vi "(SubVI)Control Data_Save or Load Control Value.vi"(5 "Val(Sgnl)":bool, 6 "Common? (f)":bool, 7 "Function":T1, 8 "error in (no error)":errorcluster caption="에러 입력(에러 없음)", 9 "Path":path, 10 "Use Default Path (t)":bool=TRUE, 11 "Control Ref":refnum<vi>[](array[refnum])) -> (0 "error out":errorcluster caption="에러 출력")   [LabVIEW 2020]
uses:
  Controls/(Ctrl)Control Data_Save or Load Control Data_Function.ctl
  Variables/(Var)System Variables.vi
  <vilib>/Utility/config.llb/Write Key (String).vi
  <vilib>/Utility/config.llb/Read Key (String).vi
  <vilib>/Utility/config.llb/NI_LVConfig.lvlib
panel:
  # "(SubVI)Save or Load Control Value.vi By hspark\n\nDescription : 컨트롤/인디케이터의 현재 값을 저장하거나, 저장된 값을 불러오는 VI\n\nInput : \n1. Control Ref : 저장 또는 불러오기를 수행할 컨트롤의 참조 배열\n2. Use Default Path : Ture 입력 시 지정된 기본 경로에 저장, False 입력 시 Path로 입력된 경로에 저장\n3. Path : Use Default Path에 False 입력 시 입력 경로 사용\n4. Function : 저장 또는 불러오기 동작 입력\n5. Val(Sgnl) : True 입력 시 값(신호) 프로퍼티로 값을 입력함 (불러오기 시에만 해당)\n6. Common?: False 입력 시 Default Path에 Chip Type을 추가한 경로 사용\n\nOutput : \n\nLabVIEW Version : 2020 SP1 이상\n\nNote :\nINI 파일 형식을 사용함\n섹션 : 컨트롤/인디케이터의 소유자 VI\n키 : 컨트롤의 라벨\n값 : 배리언트 변환 후 패턴화\n\n* 컨트롤/인디케이터 라벨 또는 VI 이름 변경 시 저장된 값 불러오기 안됨\n\nUpdate : 2022.01.06"
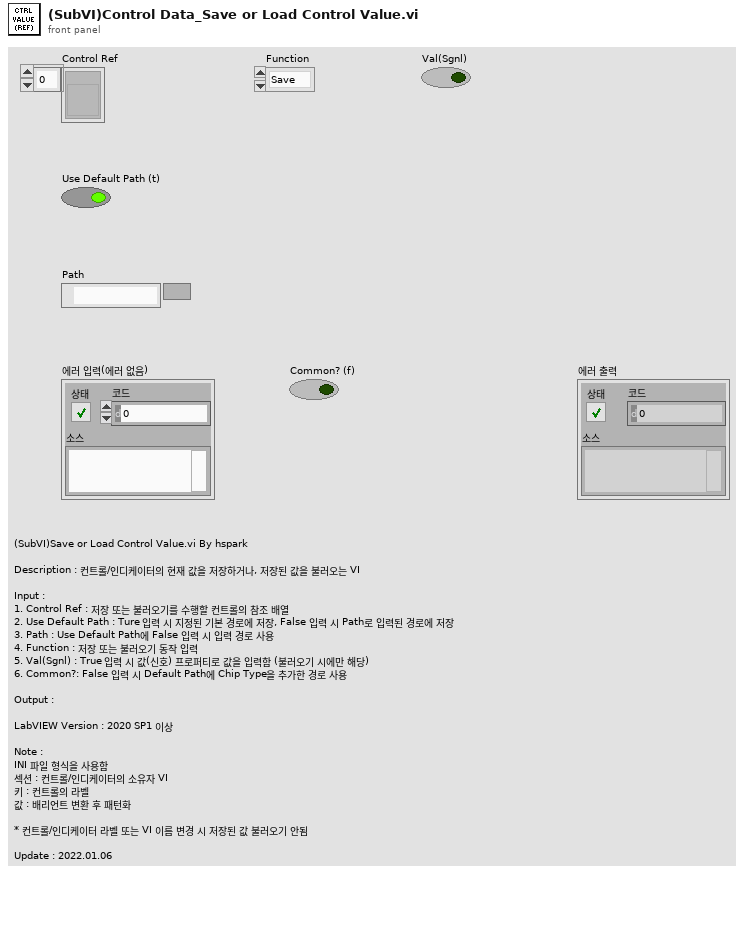
[diagram p1: front panel]
types:
  T1 = typedef "(Ctrl)Control Data_Save or Load Control Data_Function.ctl" = enum16{"Save", "Load"}
  T2 = typedef "Haptic IC.lvclass/(Ctrl)IC Type.ctl" = enum8{"DW7800", "DW7802", "DW7912", "DW7914"}
  T3 = typedef "NI_LVConfig.lvlib/Config Data RefNum.ctl" = refnum<k1>
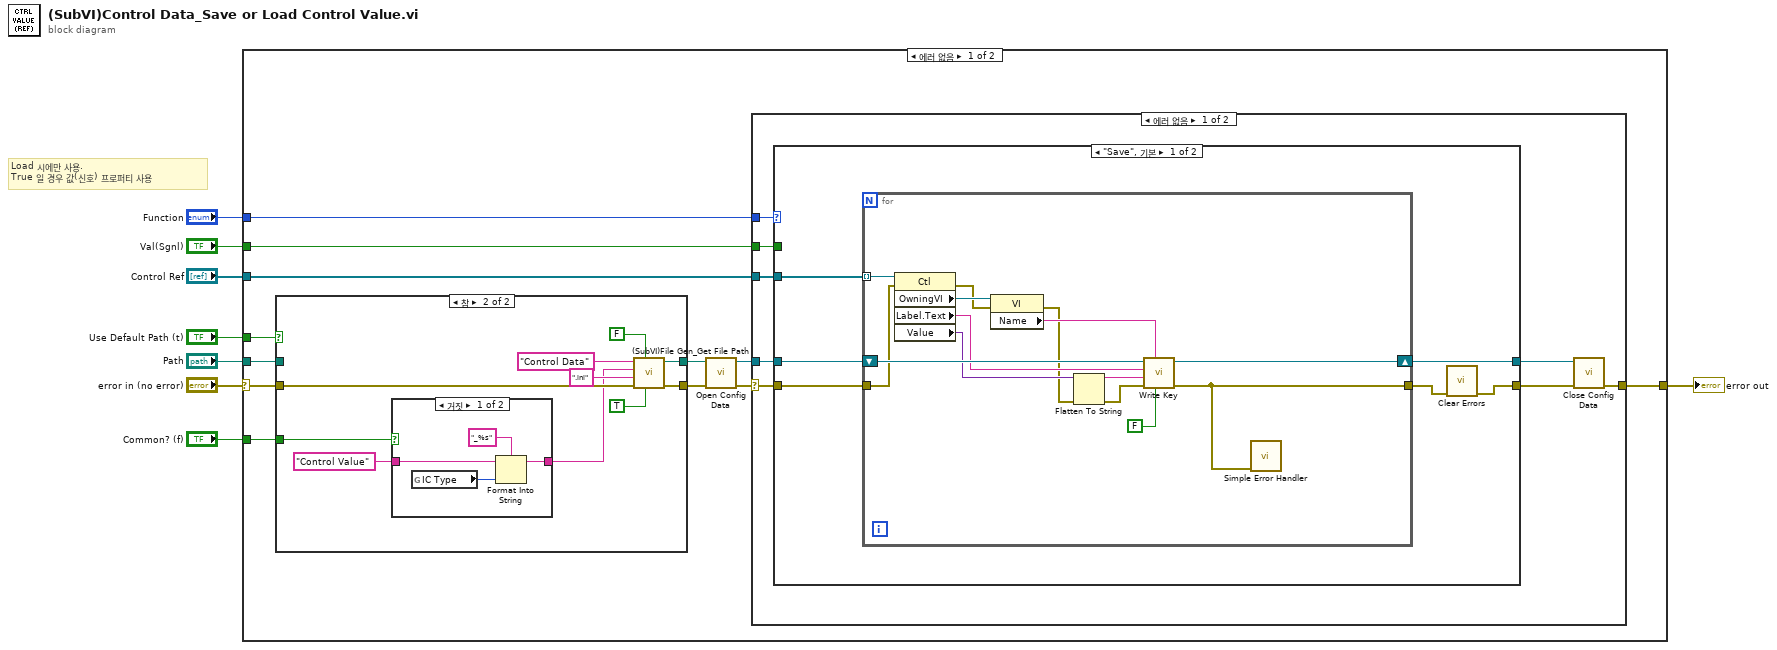
[diagram p0: block diagram]
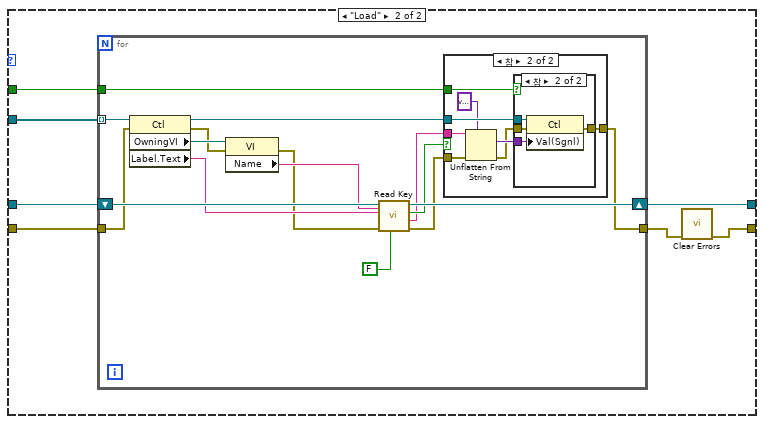
[diagram p4: hidden frame]
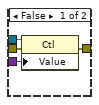
[diagram p6: hidden frame]
diagram:
  # "Load 시에만 사용.\nTrue 일 경우 값(신호) 프로퍼티 사용"
  n1 = case shown="에러 없음" "error in (no error)" {
    selector: "error in (no error)" -> [w14 w107]
    tunnel: [w18 w107] -> w7
    tunnel: "Function" -> [w17 _]
    tunnel: "Control Ref" -> [w16 _]
    tunnel: "Val(Sgnl)" -> [w15 _]
    tunnel: "Use Default Path (t)" -> [w11 _]
    tunnel: "Path" -> [w10 _]
    tunnel: "Common? (f)" -> [w9 _]
    frame No Error {
      n2 = case shown="참" w11 {
        tunnel: w14 -> [w21 w30]
        tunnel: [w21 w29] -> w13
        tunnel: [w22 w28] -> w12
        tunnel: w10 -> [w22 _]
        tunnel: w9 -> [_ w26]
        frame False {
        }
        frame True {
          n3 = case shown="거짓" w26 {
            tunnel: "Control Value" -> [w35 w37]
            tunnel: [w33 w37] -> w24
            frame False {
              n4 = global read "(Var)System Variables.vi" "IC Type"() -> (w34:T2)
              n5 = Format Into String(format string="_%s" ("포맷 문자열"), initial string=w35, w34) -> (resulting string=w33:string)  [unwired: 1 in, 1 out]
            }
            frame True {
            }
          }
          n6 = call "(SubVI)File Gen_Get File Path.vi"("Common?"=TRUE ("Common? (f)"), "Use Timestamp"=FALSE, "error in (no error)"=w30, "File Extension (.txt)"=".ini", "File Name"=w24, "Folder Name"="Control Data") -> ("error out"=w29:errorcluster, "Path"=w28:path)  [unwired: 3 in, 1 out]
        }
      }
      n7 = call <vilib>:"Open Config Data.vi"("error in (no error)"=w13, "configuration file path"=w12) -> ("error out"=w19:errorcluster, "refnum"=w20:T3)  [unwired: 7 in, 1 out]
      n8 = case shown="에러 없음" w19 {
        selector: w19 -> [w43 w106]
        tunnel: w17 -> [w45 _]
        tunnel: w20 -> [w44 _]
        tunnel: [w41 w106] -> w18
        tunnel: w16 -> [w40 _]
        tunnel: w15 -> [w38 _]
        frame No Error {
          n9 = case shown="\"Save\", 기본" w45 {
            tunnel: w44 -> [w51 w72]
            tunnel: w43 -> [w49 w70]
            tunnel: [w46 w67] -> w42
            tunnel: w40 -> [w50 w71]
            tunnel: [w48 w69] -> w39
            tunnel: w38 -> [_ w66]
            frame "Save", Default {
              n10 = for {
                tunnel: w50 -> [w65] mode=indexing
                tunnel: w49 -> [w61]
                shift-right: [w54] -> w48
                shift-left: w51 -> [w64]
                tunnel: [w52] -> w47
                n11 = property class="Ctl"(reference=w65, error in=w61) -> (error out=w62:errorcluster, "OwningVI"=w63:refnum<vi>, "Label.Text"=w59:string, "Value"=w58:variant)  [unwired: 1 out]
                n12 = property class="VI"(reference=w63, error in=w62) -> (error out=w57:errorcluster, "Name"=w60:string)  [unwired: 1 out]
                n13 = Flatten To String(anything=w58, error in (no error)=w57) -> (data string=w56:string, error out=w55:errorcluster)  [unwired: 2 in, 1 out]
                n14 = call-poly <vilib>:"Write Key.vi"("write raw string? (F)"=FALSE, "section"=w60, "error in (no error)"=w55, "value"=w56, "key"=w59, "refnum"=w64) -> ("error out"=w52:errorcluster, "refnum out"=w54:T3)  [unwired: 3 in, 1 out]
                n15 = call <vilib>:"Simple Error Handler.vi"("error in (no error)"=w52) -> ()  [unwired: 4 in, 5 out]
              }
              n16 = call <vilib>:"Clear Errors.vi"("error in (no error)"=w47) -> ("error out"=w46:errorcluster)  [unwired: 5 in, 1 out]
            }
            frame "Load" {
              n17 = for {
                tunnel: w71 -> [w88] mode=indexing
                tunnel: w70 -> [w84]
                shift-right: [w81] -> w69
                shift-left: w72 -> [w87]
                tunnel: [w73] -> w68
                tunnel: w66 -> [w74]
                n18 = property class="Ctl"(reference=w88, error in=w84) -> (reference out=w76:refnum<vi>, error out=w85:errorcluster, "OwningVI"=w86:refnum<vi>, "Label.Text"=w82:string)
                n19 = property class="VI"(reference=w86, error in=w85) -> (error out=w80:errorcluster, "Name"=w83:string)  [unwired: 1 out]
                n20 = call-poly <vilib>:"Read Key.vi"("read raw string? (F)"=FALSE ("write raw string? (F)"), "section"=w83, "error in (no error)"=w80, "key"=w82, "refnum"=w87) -> ("error out"=w75:errorcluster, "value"=w77:string, "found?"=w78:bool, "refnum out"=w81:T3)  [unwired: 3 in]
                n21 = case shown="참" w78 {
                  tunnel: w77 -> [_ w96]
                  tunnel: w76 -> [_ w97]
                  tunnel: w75 -> [w89 w93]
                  tunnel: [w89 w91] -> w73
                  tunnel: w74 -> [_ w90]
                  frame False {
                  }
                  frame True {
                    n22 = Unflatten From String(type=variant ("값"), binary string=w96, error in (no error)=w93) -> (value=w95:variant, error out=w92:errorcluster)  [unwired: 2 in, 1 out]
                    n23 = case shown="참" w90 {
                      tunnel: w97 -> [w101 w105]
                      tunnel: w95 -> [w100 w104]
                      tunnel: w92 -> [w99 w103]
                      tunnel: [w98 w102] -> w91
                      frame False {
                        n24 = property class="Ctl"(reference=w101, error in=w99, "Value"=w100) -> (error out=w98:errorcluster)  [unwired: 1 out]
                      }
                      frame True {
                        n25 = property class="Ctl"(reference=w105, error in=w103, "Val(Sgnl)"=w104) -> (error out=w102:errorcluster)  [unwired: 1 out]
                      }
                    }
                  }
                }
              }
              n26 = call <vilib>:"Clear Errors.vi"("error in (no error)"=w68) -> ("error out"=w67:errorcluster)  [unwired: 5 in, 1 out]
            }
          }
          n27 = call <vilib>:"Close Config Data.vi"("error in (no error)"=w42, "refnum"=w39) -> ("error out"=w41:errorcluster)  [unwired: 8 in, 1 out]
        }
        frame Error {
        }
      }
    }
    frame Error {
    }
  }
  "error out" <- w7
